vi "LJM logger write open configs.vi"(0 "Working Directory":path, 5 "Open Config Filename":string="LJM_Open_Any.cfg", 7 "DeviceType":string="ANY", 9 "ConnectionType":string="ANY", 11 "Identifier":string="ANY") -> (15 "error out":errorcluster)   [LabVIEW 2026]
uses:
  <vilib>/Utility/config.llb/Write Key (String).vi
  <vilib>/Utility/config.llb/NI_LVConfig.lvlib
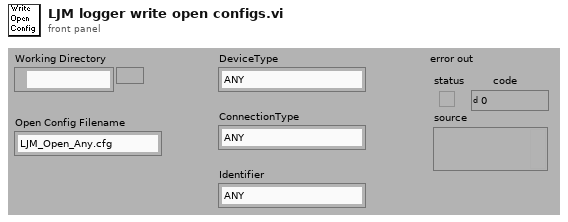
[diagram p1: front panel]
types:
  T1 = typedef "NI_LVConfig.lvlib/Config Data RefNum.ctl" = refnum<k1>
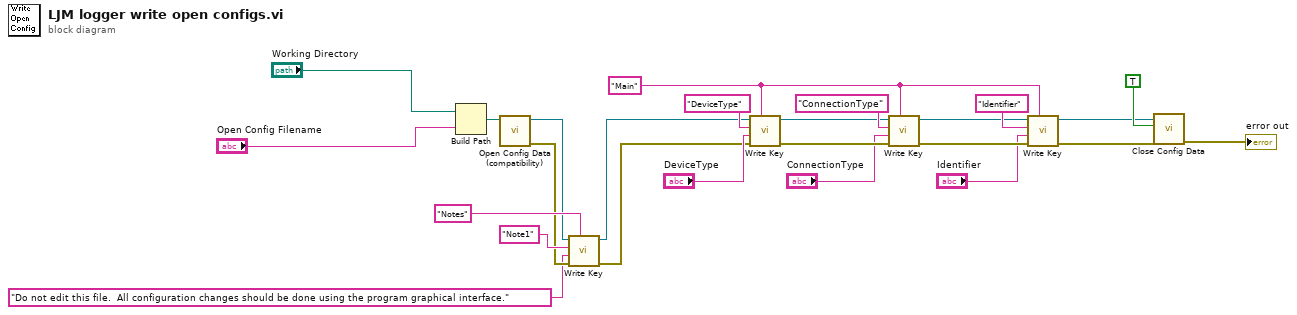
[diagram p0: block diagram]
diagram:
  w13 = "Main" ("section")
  n1 = Build Path(base path="Working Directory", name or relative path="Open Config Filename") -> (appended path=w15:path)
  n2 = call <vilib>:"Open Config Data (compatibility).vi"("configuration file path"=w15) -> ("error out"=w4:errorcluster, "refnum"=w5:T1)  [unwired: 8 in, 1 out]
  n3 = call-poly <vilib>:"Write Key.vi"("section"="Notes", "error in (no error)"=w4, "value"="Do not edit this file.  All configuration changes should be done using the program graphical interface." ("key"), "key"="Note1", "refnum"=w5) -> ("error out"=w3:errorcluster, "refnum out"=w2:T1)  [unwired: 4 in, 1 out]
  n4 = call-poly <vilib>:"Write Key.vi"("section"=w13, "error in (no error)"=w3, "value"="DeviceType", "key"="DeviceType", "refnum"=w2) -> ("error out"=w21:errorcluster, "refnum out"=w20:T1)  [unwired: 4 in, 1 out]
  n5 = call-poly <vilib>:"Write Key.vi"("section"=w13, "error in (no error)"=w21, "value"="ConnectionType", "key"="ConnectionType", "refnum"=w20) -> ("error out"=w19:errorcluster, "refnum out"=w18:T1)  [unwired: 4 in, 1 out]
  n6 = call-poly <vilib>:"Write Key.vi"("section"=w13, "error in (no error)"=w19, "value"="Identifier", "key"="Identifier", "refnum"=w18) -> ("error out"=w16:errorcluster, "refnum out"=w17:T1)  [unwired: 4 in, 1 out]
  n7 = call <vilib>:"Close Config Data.vi"("error in (no error)"=w16, "write file if changed (T)"=TRUE ("write configuration file? (F)"), "refnum"=w17) -> ("error out"=→"error out":errorcluster)  [unwired: 7 in, 1 out]
